vi "ValueSignalByPathArray.vi"(0 "VI Reference In":refnum<vi>, 5 "Control Path":string[](array[string]), 7 "Value (Signaling)":variant, 11 "error in":errorcluster) -> (4 "VI Reference Out":refnum<vi>, 15 "error out":errorcluster)   [LabVIEW 2016, in "Drona.lvlib" / "ValueSignal.lvlib"]
doc: "Sets the value of control which is specified.\n\nThe path of the control should be given in the successive index of the array"
uses:
  ValueSignal.lvlib
  Get/GetControlRef/GetControlRef.lvlib
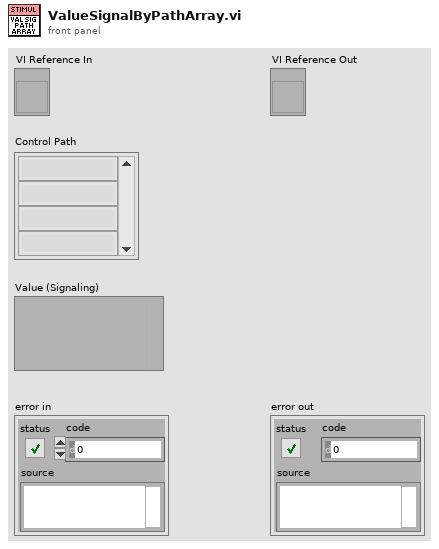
[diagram p1: front panel]
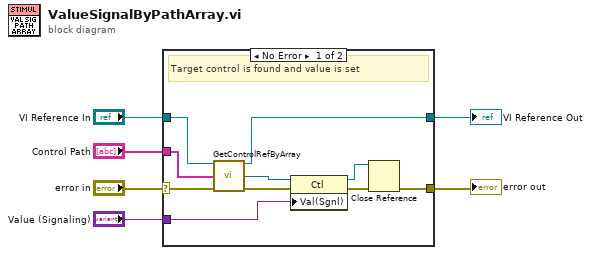
[diagram p0: block diagram]
diagram:
  n1 = case shown="No Error" "error in" {
    selector: "error in" -> [w15 w18]
    tunnel: "Control Path" -> [w12 _]
    tunnel: "VI Reference In" -> [w11 w17]
    tunnel: [w7 w17] -> w3
    tunnel: "Value (Signaling)" -> [w16 _]
    tunnel: [w10 w18] -> w1
    frame No Error {
      # "Target control is found and value is set"
      n2 = call "GetControlRefByArray.vi"("VI Reference In"=w11, "Control Path"=w12, "error In"=w15) -> ("VI Reference Out"=w7:refnum<vi>, "Ctl Refnum"=w8:refnum<vi>, "error out"=w14:errorcluster)  [unwired: 10 in]
      n3 = property class="Ctl"(reference=w8, error in=w14, "Val(Sgnl)"=w16) -> (reference out=w9:refnum<vi>, error out=w13:errorcluster)
      n4 = Close Reference(reference=w9, error in (no error)=w13) -> (error out=w10:errorcluster)
    }
    frame Error {
    }
  }
  "error out" <- w1
  "VI Reference Out" <- w3
